vi "enc_a_I64.vi"(1 "Array In":i64[](array[numeric])) -> (0 "Array Out":u8[](array[numeric]) format="%.0x")   [LabVIEW 2016, in "MsgPack.lvlib"]
uses:
  MsgPack.lvlib
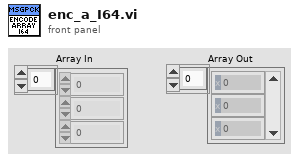
[diagram p1: front panel]
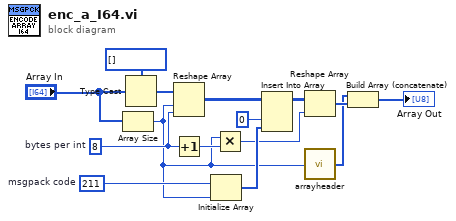
[diagram p0: block diagram]
diagram:
  w12 = u8 211  # msgpack code
  w15 = 8  # bytes per int
  n1 = Array Size(array="Array In") -> (size(s)=w6:i32)
  n2 = Type Cast(type=u8[] [], x="Array In") -> (*(type *) &x=w13:u8[])
  n3 = Reshape Array(w13, w6, w15) -> (w11:u8[][])
  n4 = Increment(x=w15) -> (x+1=w7:i32)
  n5 = Initialize Array(w12, w6) -> (w10:u8[])
  n6 = Multiply(x=w6, y=w7) -> (x*y=w5:i32)
  n7 = Insert Into Array(array=w11, index (col)=0 ("disabled index (col)"), new element=w10) -> (w9:u8[][])  [unwired: 1 in]
  n8 = Reshape Array(w9, w5) -> (w4:u8[])
  n9 = call "arrayheader.vi"("Number of Elements"=w6) -> ("header"=w3:u8[])
  n10 = Build Array (concatenate)(w3, w4) -> (→"Array Out":u8[])
